vi "GenDisplay.vi"(0 "Top Level UID ID":string, 1 "Variable Name ID":string, 3 "Data ID":string, 4 "error in (no error) ID":string, 5 "CodeParam in":refnum<class "CodeParam.lvclass">, 6 "prefix":string, 7 "Display? ID":string, 8 "app ref":refnum<vi>, 9 "Display header? (T) ID":string, 10 "Type":refnum<class "Type.lvclass">, 11 "Variable name when Display? (T) is False ID":string, 12 "Display?":bool, 13 "OutRefIdx for first node":i32=-1) -> (14 "XML":string, 18 "error out ID":string, 19 "CodeParam out":refnum<class "CodeParam.lvclass">)   [LabVIEW 2021]
uses:
  <vilib>/imath/engines/lvmath2/MathScriptCompiler/Type.llb/Type.lvclass
  <vilib>/imath/engines/lvmath2/MathScriptCompiler/CodeParam.llb/CodeParam.lvclass
  <vilib>/imath/engines/lvmath2/Utility/RunTimeEnginePaths.ctl
  <vilib>/imath/engines/lvmath2/MathScriptCompiler/Code/XML Script.llb/XML Script - Cast Type To Target RunTimeType.vi
  <vilib>/imath/engines/lvmath2/MathScriptCompiler/Type/RuntimeType.llb/RuntimeType.lvclass
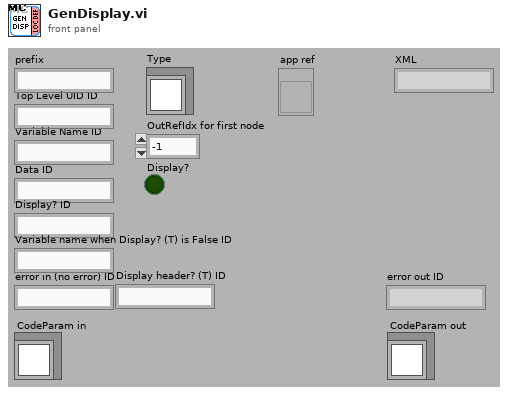
[diagram p1: front panel]
types:
  T1 = typedef "RunTimeEnginePaths.ctl" = u16
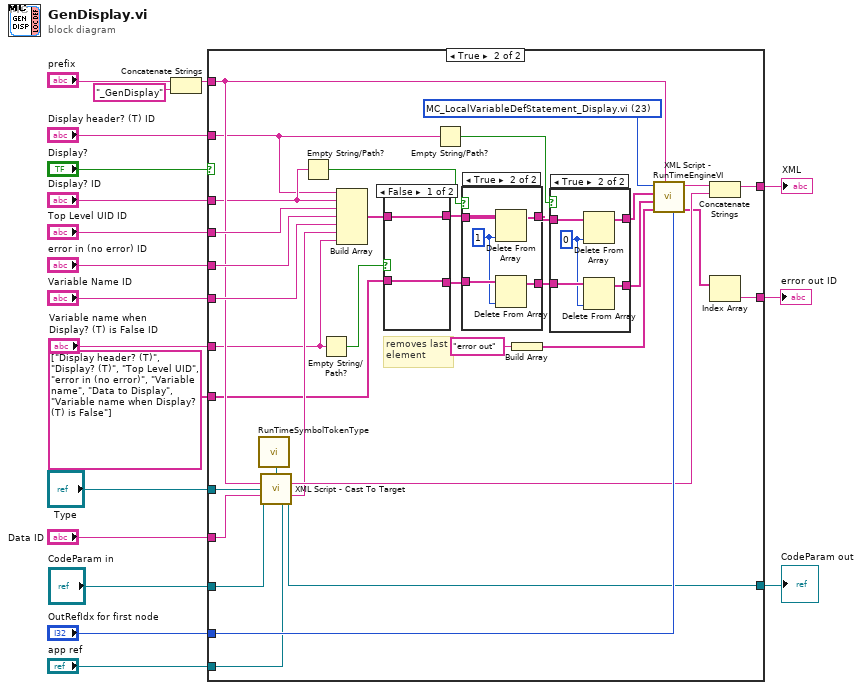
[diagram p0: block diagram]
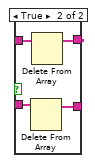
[diagram p4: hidden frame]
diagram:
  n1 = Concatenate Strings("prefix", "_GenDisplay" ("string")) -> (w6:string)
  n2 = case shown="True" "Display?" {
    tunnel: "Top Level UID ID" -> [_ w48]
    tunnel: "Data ID" -> [_ w32]
    tunnel: "Variable Name ID" -> [_ w46]
    tunnel: [_ w54] -> w15
    tunnel: "error in (no error) ID" -> [w21 w47]
    tunnel: [w21 w41] -> w19
    tunnel: "OutRefIdx for first node" -> [_ w53]
    tunnel: "Type" -> [_ w50]
    tunnel: "CodeParam in" -> [w20 w23]
    tunnel: [w20 w22] -> w9
    tunnel: w6 -> [_ w44]
    tunnel: "Variable name when Display? (T) is False ID" -> [_ w35]
    tunnel: string[] ["Display header? (T)", "Display? (T)", "Top Level UID", "error in (no error)", "Variable name", "Data to Display", "Variable name when Display? (T) is False"] -> [_ w36]
    tunnel: "Display? ID" -> [_ w33]
    tunnel: "app ref" -> [_ w31]
    tunnel: "Display header? (T) ID" -> [_ w25]
    frame False {
    }
    frame True {
      w49 = T1 23 items=["You may add additional paths to the large string constant in 'GetRunTimeEnginePath.vi', but make sure to update 'RunTimeEnginePaths.ctl' and update the default value for the array as well", "MC_ArithmeticOperator_ldivide.vi", "MC_ArithmeticOperator_minus.vi", "MC_ArithmeticOperator_mldivide.vi", "MC_ArithmeticOperator_mpower.vi", "MC_ArithmeticOperator_mrdivide.vi", "MC_ArithmeticOperator_mtimes.vi", "MC_ArithmeticOperator_plus.vi", "MC_ArithmeticOperator_power.vi", "MC_ArithmeticOperator_rdivide.vi", "MC_ArithmeticOperator_times.vi", "MC_Bitwise_Operator_And.vi", "MC_Bitwise_Operator_Not.vi", "MC_Bitwise_Operator_Or.vi", "MC_BuiltInFunction_Invoke.vi", "MC_CommandStatement_break.vi", "MC_CommandStatement_return.vi", "MC_ForEndStatement_ Index Columns.vi", "MC_ForStatement_Get Iterations.vi", "MC_IfEndStatement_SelectCase.vi", "MC_LastElement_SymbolEnd.vi", "MC_LastElement_VariableEnd.vi", "MC_LocalVariableDefStatement_Ans.vi", "MC_LocalVariableDefStatement_Display.vi", "MC_Logical_Operator.vi", "UID Generator.vi", "MC_MatrixToken_Vertcat.vi", "MC_NodeBeginStatement_Init.vi", "MC_NodeEndStatement_Dispose.vi", "MC_OverloadedArithmeticOperator_Invoke.vi", "MC_Version.vi", "MC_Range.vi", "MC_Relational_Operator_Eq.vi", "MC_Relational_Operator_Ge.vi", "MC_Relational_Operator_Gt.vi", "MC_Relational_Operator_Le.vi", "MC_Relational_Operator_Lt.vi", "MC_Relational_Operator_Ne.vi", "MC_ReplaceToken_MC,MC,MC,MC.vi", "MC_ReplaceToken_MC,MC,MC.vi", "MC_ReplaceToken_MC,MC,x,MC.vi", "MC_ReplaceToken_MC,x,MC,MC.vi", "MC_ReplaceToken_MC,x,MC.vi", "MC_ReplaceToken_MC,x,x,MC.vi", "MC_ReplaceToken_MergeChildErrors.vi", "MC_RowToken_Horzcat.vi", "MC_SymbolToken_Invoke.vi", "MathScriptCompiler_VariableDefinition.vi", "MC_VariableToken_MC,MC,MC.vi", "MC_VariableToken_MC,MC,x.vi", "MC_VariableToken_MC,MC.vi", "MC_VariableToken_MC,x,MC.vi", "MC_VariableToken_MC,x.vi", "MC_VariableToken_VariableUse.vi", "MC_Mask_Errors.vi", "MC_CommandStatement_continue.vi", "MC_pi.vi"] ("RunTimeEngine VI")
      # "removes last\nelement"
      n3 = call <vilib>:"RunTimeSymbolTokenType.vi"() -> ("RunTimeSymbolTokenType"=w52:refnum<class "RuntimeType.lvclass">)  [unwired: 1 out]
      n4 = call-poly <vilib>:"XML Script - Cast To Target.vi"("CodeParam in"=w23, "Target RunTimeType"=w52, "app ref"=w31, "prefix"=w44, "Type"=w50, "Term ID (in)"=w32) -> ("CodeParam out"=w22:refnum<class "CodeParam.lvclass">, "XML"=w51:string, "Term ID (out)"=w45:string)  [unwired: 1 in, 6 out]
      n5 = Empty String/Path?(string/path=w33) -> (empty?=w26:bool)
      n6 = Empty String/Path?(string/path=w35) -> (empty?=w34:bool)
      n7 = Build Array(w25, w33, w48, w47, w46, w45, w35) -> (w37:string[])
      n8 = case shown="False" w34 {
        tunnel: w36 -> [w63 w67]
        tunnel: w37 -> [w64 w68]
        tunnel: [w63 w66] -> w38
        tunnel: [w64 w65] -> w39
        frame False {
        }
        frame True {
          n9 = Delete From Array(array=w67) -> (array with subset deleted=w66:string[])  [unwired: 2 in, 1 out]
          n10 = Delete From Array(array=w68) -> (array with subset deleted=w65:string[])  [unwired: 2 in, 1 out]
        }
      }
      n11 = Empty String/Path?(string/path=w25) -> (empty?=w24:bool)
      n12 = case shown="True" w26 {
        tunnel: w38 -> [w69 w74]
        tunnel: w39 -> [w70 w75]
        tunnel: [w69 w73] -> w27
        tunnel: [w70 w72] -> w28
        frame False {
        }
        frame True {
          w71 = 1 ("index")
          n13 = Delete From Array(array=w75, index=w71) -> (array with subset deleted=w72:string[])  [unwired: 1 in, 1 out]
          n14 = Delete From Array(array=w74, index=w71) -> (array with subset deleted=w73:string[])  [unwired: 1 in, 1 out]
        }
      }
      n15 = Build Array("error out") -> (w42:string[])
      n16 = case shown="True" w24 {
        tunnel: w27 -> [w56 w61]
        tunnel: w28 -> [w57 w62]
        tunnel: [w56 w60] -> w29
        tunnel: [w57 w59] -> w30
        frame False {
        }
        frame True {
          w58 = 0 ("index")
          n17 = Delete From Array(array=w62, index=w58) -> (array with subset deleted=w59:string[])  [unwired: 1 in, 1 out]
          n18 = Delete From Array(array=w61, index=w58) -> (array with subset deleted=w60:string[])  [unwired: 1 in, 1 out]
        }
      }
      n19 = call <vilib>:"XML Script - RunTimeEngineVI.vi"("out"=w53, "prefix"=w44, "Output Term Names"=w42, "Input Term Names"=w29, "Input TermIDs"=w30, "RunTimeEngine VI"=w49) -> ("Output TermIDs"=w40:string[], "XML"=w55:string)  [unwired: 4 out]
      n20 = Concatenate Strings(w55, w51) -> (w54:string)
      n21 = Index Array(array=w40) -> (element=w41:string)  [unwired: 1 in]
    }
  }
  "error out ID" <- w19
  "XML" <- w15
  "CodeParam out" <- w9
